vi "pythonWriteToArrayUINT16.vi"(1 "size":i32, 2 "dst":i64, 3 "src":u16[](array[numeric])) -> (0 "dst out":i64)   [LabVIEW 2017]
uses:
  dll/wormUtilities/x64/Release/wormUtilities.dll
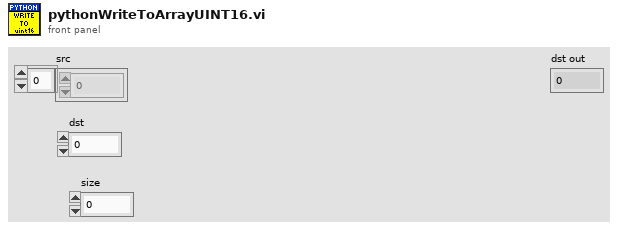
[diagram p1: front panel]
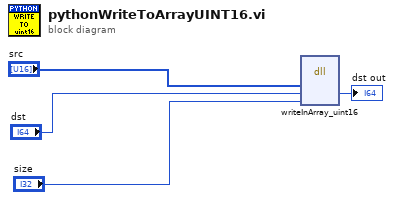
[diagram p0: block diagram]
diagram:
  n1 = dll-call lib="C:/Users/francesco/dev/pump-probe/dll/wormUtilities/x64/Release/wormUtilities.dll" fn="writeInArray_uint16"("src"="src", "dst"="dst", "size"="size") -> ("dst"=→"dst out":i64)  [unwired: 6 in, 2 out]
